vi "GE 5565PIORC.Bit Manipulation.Clear Bits (U16).vi"(8 "bit count (1)":i32=1, 9 "bit index":i32, 11 "packed value in":u16 format="%016x") -> (3 "packed value out":u16 format="%016x")   [LabVIEW 2016, in "GE 5565PIORC.lvclass"]
doc: "This VI clears the bits in the provided <B>packed value</B> starting at <B>bit index</B> and for length <B>bit count</B>."
uses:
  GE 5565PIORC.lvclass
  GE 5565PIORC.Bit Manipulation.Create Mask (U16).vi
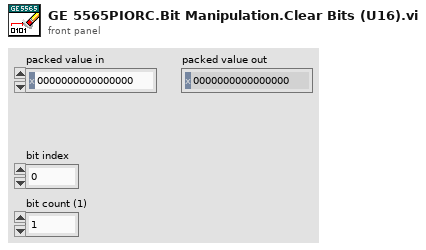
[diagram p1: front panel]
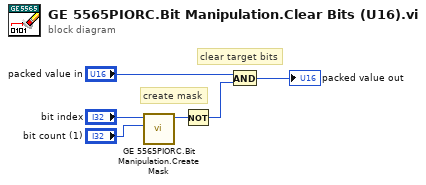
[diagram p0: block diagram]
diagram:
  # "create mask"
  # "clear target bits"
  n1 = call-poly "GE 5565PIORC.Bit Manipulation.Create Mask.vi"("bit count (1)"="bit count (1)", "bit index (0)"="bit index") -> ("mask"=w3:u16)  [unwired: 9 in]
  n2 = Not(x=w3) -> (.not. x?=w5:u16)
  n3 = And(x="packed value in", y=w5) -> (x .and. y?=→"packed value out":u16)
